vi "Contains Section.vi"(8 "error in":errorcluster, 10 "Name":string, 11 "Dictionary in":refnum<class "Dictionary.lvclass">) -> (0 "error out":errorcluster, 1 "Index":i32, 2 "Found?":bool, 3 "Dictionary out":refnum<class "Dictionary.lvclass">)   [LabVIEW 2024, in "EDS.lvlib" / "Dictionary.lvclass"]
uses:
  Dictionary.lvclass
  Dictionary.lvclass/Dictionary.ctl
  OD Section/Section.lvclass
  Section Name/Section Name.lvclass
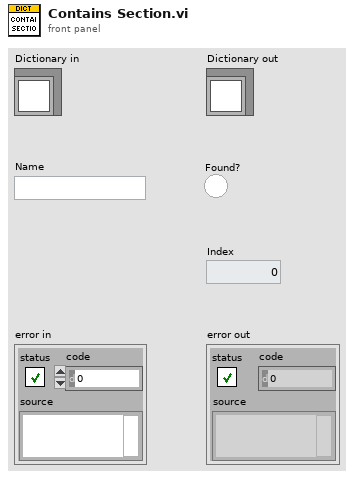
[diagram p1: front panel]
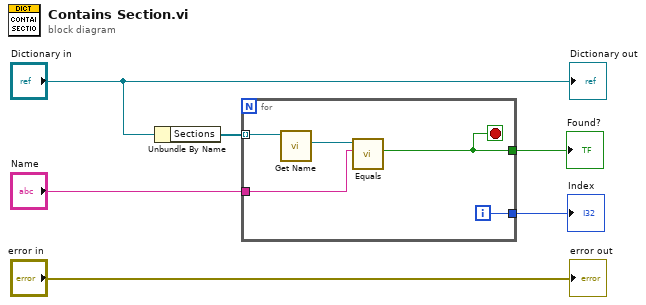
[diagram p0: block diagram]
diagram:
  n1 = Unbundle By Name("Dictionary in") -> ("Sections"=w4:refnum<class "Section.lvclass">[])
  n2 = for {
    tunnel: w4 -> [w10] mode=indexing
    tunnel: "Name" -> [w8]
    tunnel: [w11] -> w1
    tunnel: [w7] -> w2
    i -> [w11]
    stop <- w7 stop-if-true
    n3 = call "Get Name.vi"("Object Entry in"=w10) -> ("Section Name"=w9:refnum<class "Section Name.lvclass">)  [unwired: 9 in, 1 out]
    n4 = call "Equals.vi"("String"=w8, "Section Name in"=w9) -> ("Equal?"=w7:bool)  [unwired: 8 in, 1 out]
  }
  "Found?" <- w2
  "Index" <- w1
  "error out" <- "error in"
  "Dictionary out" <- "Dictionary in"
